vi "Overwrite Physical Channel.vi"(8 "error in (no error)":errorcluster, 9 "Index":i32, 10 "DAQmx Physical Channel":tag, 11 "Instrument Specifications in":T1) -> (0 "error out":errorcluster, 3 "Instrument Specifications out":T1)   [LabVIEW 2026, in "Settings.lvlib"]
uses:
  Settings.lvlib
  Acquisition/Instrument Specifications Configuration.ctl
  Acquisition/Instrument Specifications Cluster Configuration.ctl
  controls/UI/Measurement Role.ctl
  Acquisition/Acquisition.lvlib
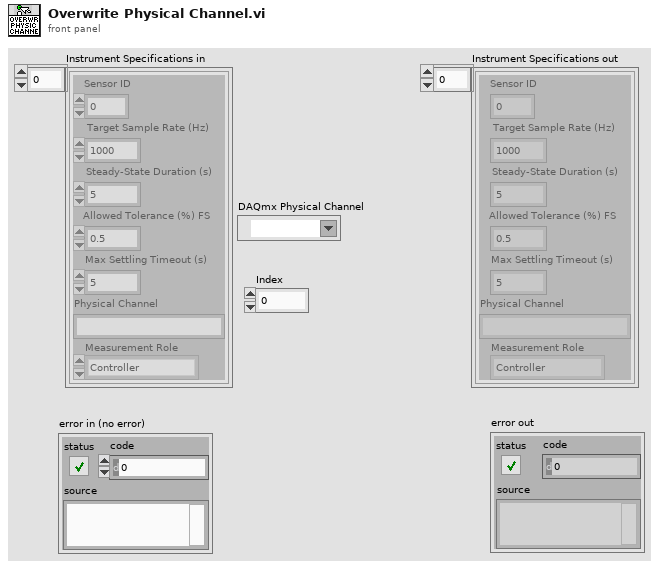
[diagram p1: front panel]
types:
  T1 = typedef "Acquisition.lvlib/Instrument Specifications Configuration.ctl" = T2[]
  T2 = typedef "Acquisition.lvlib/Instrument Specifications Cluster Configuration.ctl" = cluster{"Sensor ID":i32, "Target Sample Rate (Hz)":dbl, "Steady-State Duration (s)":i32, "Allowed Tolerance (%) FS":dbl, "Max Settling Timeout (s)":i32, "Physical Channel":string, "Measurement Role":T3}
  T3 = typedef "Settings.lvlib/Measurement Role.ctl" = enum16{"Controller", "Reference", "UUT", "Disable", "All"}
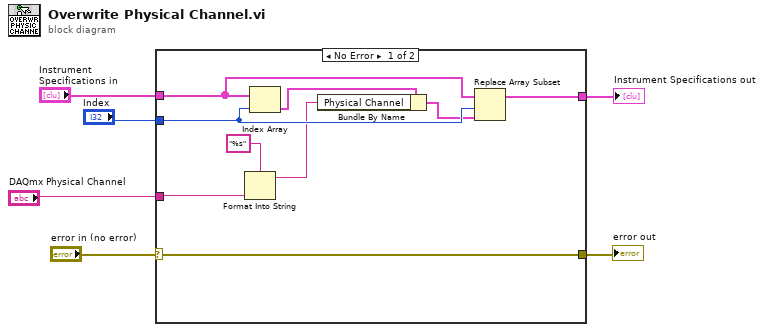
[diagram p0: block diagram]
diagram:
  n1 = case shown="No Error" "error in (no error)" {
    selector: "error in (no error)" -> [w12 w17]
    tunnel: [w15 w16] -> w6
    tunnel: "Index" -> [w14 _]
    tunnel: "Instrument Specifications in" -> [w13 w16]
    tunnel: [w12 w17] -> w2
    tunnel: "DAQmx Physical Channel" -> [w9 _]
    frame No Error {
      n2 = Format Into String(format string="%s", w9) -> (resulting string=w8:string)  [unwired: 2 in, 1 out]
      n3 = Index Array(array=w13, index=w14) -> (element=w10:T2)
      n4 = Bundle By Name(cluster=w10, "Physical Channel"=w8) -> (w11:T2)
      n5 = Replace Array Subset(array=w13, new element=w11, index=w14) -> (w15:T1)
    }
    frame Error {
    }
  }
  "Instrument Specifications out" <- w6
  "error out" <- w2
